vi "boolean to bit string.vi"() -> ()   [LabVIEW 2020]
panel:
  out "data string 2":string
  out "data string":string
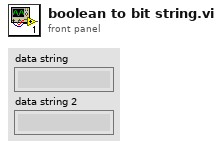
[diagram p1: front panel]
types:
  T1 = cluster{bool, bool, bool, bool, bool, bool, bool, bool}
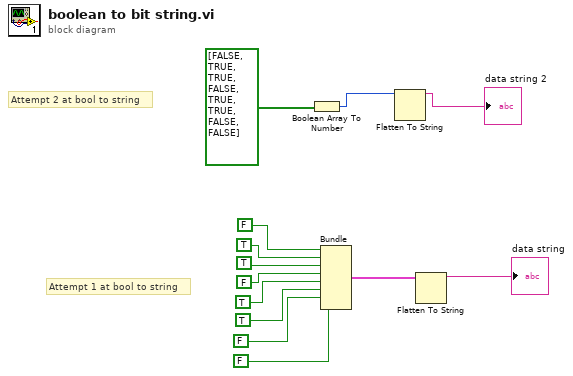
[diagram p0: block diagram]
diagram:
  # "Attempt 2 at bool to string"
  # "Attempt 1 at bool to string"
  n1 = Boolean Array To Number(Boolean array=bool[] [FALSE, TRUE, TRUE, FALSE, TRUE, TRUE, FALSE, FALSE]) -> (number=w1:u32)
  n2 = Bundle(FALSE, TRUE, TRUE, FALSE, TRUE, TRUE, FALSE, FALSE) -> (w12:T1)  [unwired: 1 in]
  n3 = Flatten To String(anything=w1) -> (data string=→"data string 2":string)  [unwired: 3 in, 2 out]
  n4 = Flatten To String(anything=w12) -> (data string=→"data string":string)  [unwired: 3 in, 2 out]
